vi "Video feed info class VI - retrieve video info.vi"(0 "Video feed info in":refnum<class "Video feed info.lvclass">, 11 "error in (no error)":errorcluster) -> (2 "file path":path, 3 "Avi Refnum (duplicate)":T1, 4 "Video feed info out":refnum<class "Video feed info.lvclass">, 6 "Image Type":T2 items=["Grayscale (U8)", "Grayscale (I16)", "Grayscale (SGL)", "Complex (CSG)", "RGB (U32)", "HSL (U32)", "RGB (U64)", "Grayscale (U16)"], 8 "height":u32, 10 "width":u32, 13 "FPS":u32, 14 "Number of Frames":u32, 15 "error out":errorcluster)   [LabVIEW 2010, in "Video feed info.lvclass"]
uses:
  Video feed info.lvclass
  <vilib>/vision/Avi1.llb/AviRefnum.ctl
  Video feed info.lvclass/Video feed info.ctl
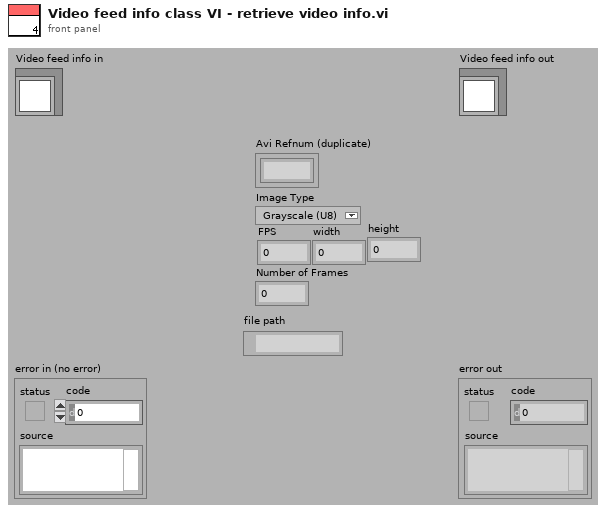
[diagram p1: front panel]
types:
  T1 = typedef "AviRefnum.ctl" = refnum<k1>
  T2 = typedef "Image Type" = u32
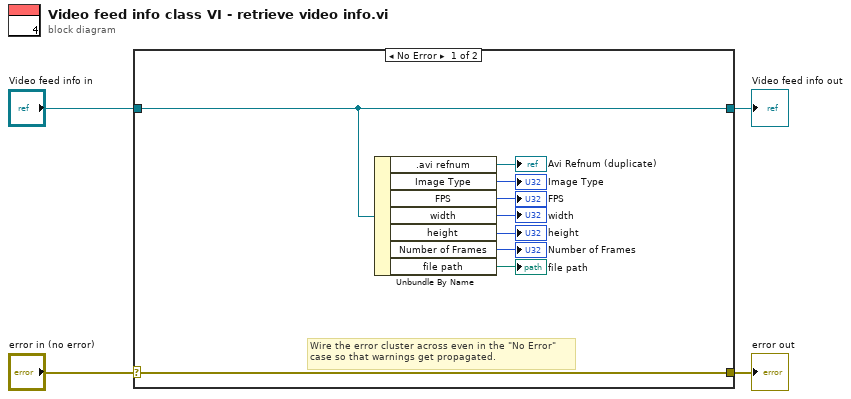
[diagram p0: block diagram]
diagram:
  n1 = case shown="No Error" "error in (no error)" {
    selector: "error in (no error)" -> [w13 w15]
    tunnel: [w13 w15] -> w3
    tunnel: [w12 w14] -> w1
    tunnel: "Video feed info in" -> [w12 w14]
    frame No Error {
      # "Wire the error cluster across even in the \"No Error\"\ncase so that warnings get propagated."
      n2 = Unbundle By Name(w12) -> (".avi refnum"=→"Avi Refnum (duplicate)":T1, "Image Type"=→"Image Type":T2, "FPS"=→"FPS":u32, "width"=→"width":u32, "height"=→"height":u32, "Number of Frames"=→"Number of Frames":u32, "file path"=→"file path":path)
    }
    frame Error {
    }
  }
  "error out" <- w3
  "Video feed info out" <- w1
